vi "纳清_清扫模式.vi"(7 "探头":u16(ring) items=["null", "pH", "DO", "浊度", "电导率", "叶绿素a", "藻密度"], 8 "error in (no error)":errorcluster caption="错误输入（无错误）", 11 "清扫模式":u16(ring)=1 items=["自动清扫", "手动清扫", "启动一次清扫"]) -> (0 "error out":errorcluster caption="错误输出")   [LabVIEW 2016, in "斯坦道多参数.lvlib"]
uses:
  <vilib>/Plasmionique/MB Master/MB_Master/MB_Master.lvclass
  <vilib>/Plasmionique/MB Master/MB Master.lvlib
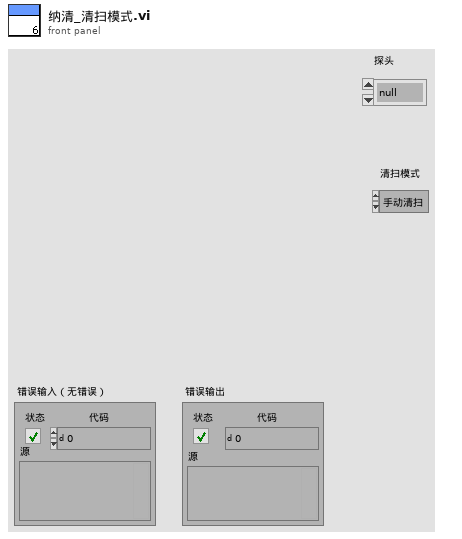
[diagram p1: front panel]
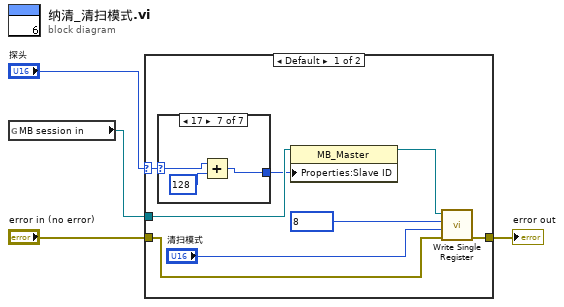
[diagram p0: block diagram]
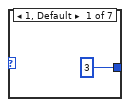
[diagram p2: hidden frame]
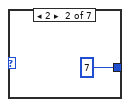
[diagram p3: hidden frame]
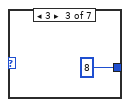
[diagram p4: hidden frame]
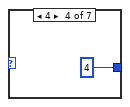
[diagram p5: hidden frame]
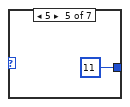
[diagram p6: hidden frame]
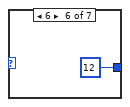
[diagram p7: hidden frame]
diagram:
  n1 = global read "多参数全局变量.vi" "MB session in"() -> (w1:refnum<class "MB_Master.lvclass">)
  n2 = case shown="Default" "探头" {
    selector: "探头" -> [w10 _]
    tunnel: "error in (no error)" -> [w9 w22]
    tunnel: [w5 w22] -> w3
    tunnel: w1 -> [w12 _]
    frame Default {
      n3 = case shown="17" w10 {
        selector: w10 -> [_ _ _ _ _ _ w21]
        tunnel: [3 7 8 4 11 12 w19] -> w11
        frame 1, Default {
        }
        frame 2 {
        }
        frame 3 {
        }
        frame 4 {
        }
        frame 5 {
        }
        frame 6 {
        }
        frame 17 {
          n4 = Add(x=w21, y=u16 128) -> (x+y=w19:u16)
        }
      }
      n5 = property class="MB_Master"(reference=w12, "Properties:Slave ID"=w11) -> (reference out=w8:refnum<class "MB_Master.lvclass">)  [unwired: 1 in, 1 out]
      n6 = call <vilib>:"Write Single Register.vi"("error in (no error)"=w9, "value"="清扫模式", "address"=u16 8 ("starting address"), "MB session in"=w8) -> ("error out"=w5:errorcluster)  [unwired: 6 in, 1 out]
    }
    frame 0 {
    }
  }
  "error out" <- w3
